vi "UNITEST MAIN v2.0.vi"() -> ()   [LabVIEW 2025] (continued)
    n868 = Close Reference(reference=w1021, error in (no error)=w1022) -> ()  [unwired: 1 out]
    n869 = Equal?(x=w1020, y=TRUE) -> (x = y?=w1018:bool)
    n870 = Select(t=i64 10 ("Period"), s=w1018, f=i64 100) -> (s? t:f=w1014:i64)
    n871 = Wait Until Next ms Multiple(millisecond multiple=w1014) -> ()  [unwired: 1 out]
  }
  n872 = timed-loop "Timed Loop" {
    shift-right: [w1107] -> _
    shift-left: w9 -> [w1108]
    tunnel: [w1101] -> w12
    tunnel: w41 -> [w1099]
    tunnel: w6 -> [w1098]
    tunnel: w10 -> [w1097]
    timing: w26 -> [_]
    timing-out: [_] -> w25
    shift-right: [w1095] -> _
    shift-left: w24 -> [w1096]
    shift-right: [w1093] -> _
    shift-left: w24 -> [w1094]
    shift-right: [w1091] -> _
    shift-left: w24 -> [w1092]
    shift-right: [w1090] -> _
    shift-left: w24 -> [w1089]
    stop <- w1106 stop-if-true
    # "Load Pid  Handling Loop"
    n873 = node-c288() -> ()  [unwired: 1 in, 1 out]
    n874 = call "Dequeue Message.vi"("error in (no error)"=w1098, "Message Queue"=w1099) -> ("error out"=w1105:errorcluster, "Message Data"=w1103:variant, "Message"=w1104:string, "dup Message Queue"=w1102:refnum<queue>)  [unwired: 6 in]
    n875 = case "Message Cases" shown="\"Load Pid Main\"" w1104 {
      selector: w1104 -> [_ _ _ _ _ w1216]
      tunnel: w1102 -> [w1115 w1144 _ w1195 w1211 _]
      tunnel: w1105 -> [w1118 w1142 w1188 w1199 w1205 _]
      tunnel: [w1119 w1145 w1182 w1197 w1207 w1217] -> w1100
      tunnel: w1108 -> [w1117 w1131 w1187 w1198 w1210 w1218]
      tunnel: [w1117 w1131 w1187 w1198 w1210 w1218] -> w1107
      tunnel: [_ _ _ _ TRUE _] -> w1106
      tunnel: w1103 -> [_ _ w1186 _ _ _]
      tunnel: w1097 -> [_ _ _ _ w1204 _]
      tunnel: w1096 -> [w1113 w1127 w1181 w1192 w1203 w1214]
      tunnel: [w1113 w1126 w1181 w1192 w1203 w1214] -> w1095
      tunnel: w1094 -> [w1114 w1125 w1180 w1191 w1202 w1215]
      tunnel: [w1114 w1124 w1180 w1191 w1202 w1215] -> w1093
      tunnel: w1092 -> [w1112 w1123 w1179 w1190 w1201 w1213]
      tunnel: [w1112 w1122 w1179 w1190 w1201 w1213] -> w1091
      tunnel: w1089 -> [_ w1121 _ _ _ _]
      tunnel: [w1111 w1120 w1178 w1189 w1200 w1212] -> w1090
      tunnel: w1089 -> [w1111 _ w1178 w1189 w1200 w1212]
      frame "init" {
        # "Initialize - All initialization work should take place in this message, since other loops can potentially enqueue messages that execute immediately after this one."
        n876 = call-poly "Enqueue Message.vi"("error in (no error)"=w1118, "Message"="Load Pid Main", "Message Queue"=w1115) -> ("error out"=w1119:errorcluster)  [unwired: 7 in, 1 out]
      }
      frame "Load Pid Main" {
        n877 = Unbundle By Name(w1131) -> ("Main Screen.Load En"=w1137:refnum<vi>)
        n878 = Unbundle By Name(w1131) -> ("PID.apply load"=w1132:refnum<vi>)
        n879 = property on="Property Node" class="Bool (strict)"(reference=w1137) -> (reference out=w1135:refnum<vi>, error out=w1136:errorcluster, "Value"=w1130:bool)  [unwired: 1 in]
        n880 = property on="Property Node" class="Bool (strict)"(reference=w1132) -> (reference out=w1134:refnum<vi>, error out=w1133:errorcluster, "Value"=w1129:bool)  [unwired: 1 in]
        n881 = Close Reference(reference=w1135, error in (no error)=w1136) -> ()  [unwired: 1 out]
        n882 = Close Reference(reference=w1134, error in (no error)=w1133) -> ()  [unwired: 1 out]
        n883 = Or(x=w1130, y=w1129) -> (x .or. y?=w1128:bool)
        n884 = case shown="True" w1128 {
          tunnel: w1142 -> [w1152 w1165]
          tunnel: [w1152 w1164] -> w1138
          tunnel: w1131 -> [_ w1163]
          tunnel: w1127 -> [w1151 w1162]
          tunnel: [w1151 w1161] -> w1126
          tunnel: w1125 -> [w1150 w1160]
          tunnel: [w1150 w1159] -> w1124
          tunnel: w1123 -> [w1147 w1156]
          tunnel: [w1147 w1155] -> w1122
          tunnel: w1121 -> [w1146 w1154]
          tunnel: [w1146 w1153] -> w1120
          frame False {
            n885 = local write "Checkbox 2"(TRUE ("Checkbox 2")) -> ()
            n886 = local write "Checkbox"(TRUE ("Checkbox")) -> ()
          }
          frame True {
            n887 = case shown="True" "Checkbox 2" {
              selector: "Checkbox 2" -> [_ w1168]
              tunnel: [FALSE ("Checkbox") "Checkbox"] -> w1158
              frame False {
              }
              frame True {
                n888 = Not(x=w1168) -> (.not. x?=w1167:bool)
                n889 = local write "Checkbox 2"(w1167) -> ()
              }
            }
            n890 = call "NEW LOAD CELL PID.vi"("filtered_load_in"=w1156, "filtered_deriv_in"=w1154, "integral_out"=w1160, "error in (no error)"=w1165, "prev_error_out"=w1162, "Checkbox"=w1158, "main ref"=w1163) -> ("error out"=w1164:errorcluster, "prev_error_out"=w1161:dbl, "integral_out"=w1159:dbl, "filtered_load_out"=w1155:dbl, "filtered_deriv_out"=w1153:dbl)
          }
        }
        n891 = Unbundle By Name(w1131) -> ("Main Home Screen.EXIT"=w1143:refnum<vi>)
        n892 = property on="Property Node" class="Bool (strict)"(reference=w1143) -> (reference out=w1140:refnum<vi>, error out=w1141:errorcluster, "Value"=w1139:bool)  [unwired: 1 in]
        n893 = case shown="False" w1139 {
          tunnel: [w1172 w1176] -> w1145
          tunnel: w1144 -> [w1171 w1175]
          tunnel: w1138 -> [w1170 w1174]
          frame True {
            n894 = call-poly "Enqueue Message.vi"("error in (no error)"=w1170, "Message"="Confirm Quit", "Message Queue"=w1171) -> ("error out"=w1172:errorcluster)  [unwired: 7 in, 1 out]
          }
          frame False {
            n895 = call-poly "Enqueue Message.vi"("error in (no error)"=w1174, "Message"="Load Pid Main", "Message Queue"=w1175) -> ("error out"=w1176:errorcluster)  [unwired: 7 in, 1 out]
          }
        }
        n896 = Close Reference(reference=w1140, error in (no error)=w1141) -> ()  [unwired: 1 out]
      }
      frame "Error" {
        # "#CodeRecommended - If you ever change the name of this \"Error\" message, you'll need to update the name in the Check Loop Error.vi as well."
        # "#CodeRecommended - Consider creating a system for logging errors in some way. These errors are for notification purposes only. Handling of specific errors should be performed in the message frames that generated the error."
        # "Error - Display an error dialog. This message is sent by the \"Error Handler\" VIs at the end of other loops in this application."
        n897 = Variant To Data(error in=w1188, type=errorcluster {"status"=FALSE, "code"=0, "source"=""} ("error constant"), Variant=w1186) -> (data=w1184:errorcluster, error out=w1183:errorcluster)
        n898 = call <vilib>:"Simple Error Handler.vi"("error in (no error)"=w1184) -> ()  [unwired: 4 in, 5 out]
        n899 = Merge Errors(w1183) -> (w1182:errorcluster)
      }
      frame "Confirm Quit" {
        # "#CodeNeeded - If you want to provide an \"Are you sure\" dialog (or some other notification) before the application exits, place that code here. This message is typically sent from a Panel Close? event."
        # "Confirm Quit - Message that can confirm whether or not the user wants to exit the application."
        n900 = call-poly "Enqueue Message.vi"("Priority Message? (F)"=TRUE, "error in (no error)"=w1199, "Message"="Exit", "Message Queue"=w1195) -> ("error out"=w1196:errorcluster)  [unwired: 6 in, 1 out]
        n901 = Merge Errors(w1196) -> (w1197:errorcluster)
      }
      frame "Exit" {
        # "Stop the VI"
        # "Release the message queue reference"
        # "#CodeNeeded - Add any required cleanup code here. Note that if 'Exit' was called as a result of an error, an error dialog will be displayed. Add any custom error handling for an 'Exit' condition here as well."
        # "Exit - Exit the application."
        n902 = call "Fire User Event - Stop.vi"("User Event - Stop"=w1204) -> ("error out"=w1206:errorcluster)  [unwired: 10 in]
        n903 = Release Queue(queue=w1211, error in (no error)=w1205) -> (error out=w1208:errorcluster)  [unwired: 1 in, 2 out]
        n904 = Merge Errors(w1206, w1208) -> (w1207:errorcluster)
      }
      frame Default {
        # "'Default' case only runs if there is a message that isn't defined in any of the other cases.  Output a programming error."
        n905 = xnode ("Error Ring")("parameter 0"=w1216) -> ("error out"=w1217:errorcluster)
      }
    }
    n906 = call "LAB-IQ Error Handler - Message Handling Loop.vi"("error in (no error)"=w1100, "Message Queue"=w1102) -> ("dup error in"=w1101:errorcluster)  [unwired: 8 in, 1 out]
    n907 = node-c288() -> ()  [unwired: 1 in, 1 out]
  }
  n908 = timed-loop {
    shift-right: [w1228] -> _
    shift-left: w9 -> [w1253]
    tunnel: [w1247] -> w5
    tunnel: w7 -> [w1245]
    tunnel: w6 -> [w1244]
    tunnel: w10 -> [w1243]
    timing: w4 -> [_]
    timing-out: [_] -> w3
    stop <- w1252 stop-if-true
    # "Acqoustic  Handling Loop"
    n909 = node-c288() -> ()  [unwired: 1 in, 1 out]
    n910 = call "Dequeue Message.vi"("error in (no error)"=w1244, "Message Queue"=w1245) -> ("error out"=w1251:errorcluster, "Message Data"=w1249:variant, "Message"=w1250:string, "dup Message Queue"=w1248:refnum<queue>)  [unwired: 6 in]
    n911 = case "Message Cases" shown="\"init\"" w1250 {
      selector: w1250 -> [_ _ _ _ _ w1350]
      tunnel: w1248 -> [w1268 w1283 _ w1337 w1349 _]
      tunnel: w1251 -> [w1262 w1274 w1334 w1341 w1343 _]
      tunnel: [w1270 w1284 w1328 w1339 w1345 w1351] -> w1246
      tunnel: w1253 -> [w1259 w1273 w1333 w1340 w1348 w1352]
      tunnel: [w1259 w1273 w1333 w1340 w1348 w1352] -> w1228
      tunnel: [_ _ _ _ TRUE _] -> w1252
      tunnel: w1249 -> [_ _ w1332 _ _ _]
      tunnel: w1243 -> [_ _ _ _ w1342 _]
      frame "init" {
        (unwired) dbl[] [] ("0UTPUT")
        # "Initialize - All initialization work should take place in this message, since other loops can potentially enqueue messages that execute immediately after this one."
        n912 = call "Acq Write Loop.vi"("Enum - Menu"=Write_Main_Enum."INIT", "error in (no error)"=w1262, "main ref"=w1259) -> ("error out"=w1267:errorcluster)  [unwired: 8 in]
        n913 = call <vilib>:"Clear Errors.vi"("error in (no error)"=w1267) -> ("error out"=w1266:errorcluster)  [unwired: 5 in, 1 out]
        n914 = call "Stall Data Flow.vim"("value in"=w1266, "milliseconds to wait"=u32 1000) -> ("value out"=w1265:errorcluster)  [unwired: 1 out]
        n915 = call "Acq Read Loop.vi"("Enum - Menu"=Read_Main_Enum."INIT", "error in (no error)"=w1265, "main ref"=w1259) -> ("error out"=w1263:errorcluster)  [unwired: 7 in, 1 out]
        n916 = call <vilib>:"Clear Errors.vi"("error in (no error)"=w1263) -> ("error out"=w1261:errorcluster)  [unwired: 5 in, 1 out]
        n917 = call-poly "Enqueue Message.vi"("error in (no error)"=w1261, "Message"="Acoustic Main", "Message Queue"=w1268) -> ("error out"=w1270:errorcluster)  [unwired: 7 in, 1 out]
      }
      frame "Acoustic Main" {
        n918 = Unbundle By Name(w1273) -> ("Environmental control.Acoustic Emission 3"=w1278:refnum<vi>)
        n919 = property on="Property Node" class="Bool (strict)"(reference=w1278) -> (reference out=w1276:refnum<vi>, error out=w1277:errorcluster, "Value"=w1275:bool)  [unwired: 1 in]
        n920 = Close Reference(reference=w1276, error in (no error)=w1277) -> ()  [unwired: 1 out]
        n921 = case shown="True" w1275 {
          tunnel: w1274 -> [w1285 w1315]
          tunnel: w1273 -> [_ w1287]
          tunnel: [w1285 w1307] -> w1272
          frame False {
          }
          frame True {
            n922 = call "Acq Read Loop.vi"("Enum - Menu"=Read_Main_Enum."READ", "error in (no error)"=w1315, "main ref"=w1287) -> ("error out"=w1313:errorcluster, "ERROR TEMP"=w1312:bool)  [unwired: 7 in]
            n923 = Unbundle By Name(w1287) -> ("Acquostic.Downlink Packet"=w1311:refnum<vi>)
            n924 = case shown="False" w1312 {
              tunnel: w1313 -> [w1316 w1319]
              tunnel: [w1316 w1318] -> w1308
              tunnel: w1287 -> [_ w1317]
              frame False {
              }
              frame True {
                n925 = call "Acoustic Reinitize.vi"("error in (no error)"=w1319, "Data Cluster"=w1317) -> ("error out"=w1318:errorcluster)  [unwired: 9 in]
              }
            }
            n926 = property on="Property Node" class="Clust (strict)"(reference=w1311, error in=w1308) -> (reference out=w1309:refnum<vi>, error out=w1310:errorcluster, "Value"=w1293:T8)
            n927 = Close Reference(reference=w1309, error in (no error)=w1310) -> (error out=w1307:errorcluster)
            n928 = Unbundle By Name(w1293) -> ("AE Ring-Down Counts"=w1291:u32)
            n929 = Unbundle By Name(w1293) -> ("Amplitude dB_AE"=w1292:sgl)
            n930 = Unbundle By Name(w1293) -> ("Peak Amplitude"=w1297:sgl)
            n931 = Unbundle By Name(w1293) -> ("Signal Energy"=w1286:sgl)
            n932 = Unbundle By Name(w1287) -> ("Main Screen.Acoustic Emission (mV)"=w1289:refnum<vi>)
            n933 = Unbundle By Name(w1287) -> ("Acquostic.Signal Energy"=w1306:refnum<vi>)
            n934 = Unbundle By Name(w1287) -> ("Acquostic.Amplitude db_AE"=w1301:refnum<vi>)
            n935 = Unbundle By Name(w1287) -> ("Acquostic.Peak Amplitude"=w1300:refnum<vi>)
            n936 = Unbundle By Name(w1287) -> ("Acquostic.AE Ring-Down Counts"=w1294:refnum<vi>)
            n937 = property class="DigNum (strict)"(reference=w1289, "Value"=w1286) -> (reference out=w1288:refnum<vi>, error out=w1290:errorcluster)  [unwired: 1 in]
            n938 = property on="Property Node" class="WFChart (strict)"(reference=w1306, "Value"=w1286) -> (reference out=w1304:refnum<vi>, error out=w1305:errorcluster)  [unwired: 1 in]
            n939 = property on="Property Node" class="WFChart (strict)"(reference=w1301, "Value"=w1292) -> (reference out=w1303:refnum<vi>, error out=w1302:errorcluster)  [unwired: 1 in]
            n940 = property on="Property Node" class="WFChart (strict)"(reference=w1300, "Value"=w1297) -> (reference out=w1298:refnum<vi>, error out=w1299:errorcluster)  [unwired: 1 in]
            n941 = property on="Property Node" class="WFChart (strict)"(reference=w1294, "Value"=w1291) -> (reference out=w1296:refnum<vi>, error out=w1295:errorcluster)  [unwired: 1 in]
            n942 = Close Reference(reference=w1288, error in (no error)=w1290) -> ()  [unwired: 1 out]
            n943 = Close Reference(reference=w1304, error in (no error)=w1305) -> ()  [unwired: 1 out]
            n944 = Close Reference(reference=w1303, error in (no error)=w1302) -> ()  [unwired: 1 out]
            n945 = Close Reference(reference=w1298, error in (no error)=w1299) -> ()  [unwired: 1 out]
            n946 = Close Reference(reference=w1296, error in (no error)=w1295) -> ()  [unwired: 1 out]
          }
        }
        n947 = Unbundle By Name(w1273) -> ("Main Home Screen.EXIT"=w1282:refnum<vi>)
        n948 = property on="Property Node" class="Bool (strict)"(reference=w1282) -> (reference out=w1280:refnum<vi>, error out=w1281:errorcluster, "Value"=w1279:bool)  [unwired: 1 in]
        n949 = call <vilib>:"Clear Errors.vi"("error in (no error)"=w1272) -> ("error out"=w1271:errorcluster)  [unwired: 5 in, 1 out]
        n950 = Close Reference(reference=w1280, error in (no error)=w1281) -> ()  [unwired: 1 out]
        n951 = case shown="False" w1279 {
          tunnel: [w1322 w1326] -> w1284
          tunnel: w1283 -> [w1321 w1325]
          tunnel: w1271 -> [w1320 w1324]
          frame True {
            n952 = call-poly "Enqueue Message.vi"("error in (no error)"=w1320, "Message"="Confirm Quit", "Message Queue"=w1321) -> ("error out"=w1322:errorcluster)  [unwired: 7 in, 1 out]
          }
          frame False {
            n953 = call-poly "Enqueue Message.vi"("error in (no error)"=w1324, "Message"="Acoustic Main", "Message Queue"=w1325) -> ("error out"=w1326:errorcluster)  [unwired: 7 in, 1 out]
          }
        }
      }
      frame "Error" {
        (unwired) dbl[] [] ("0UTPUT")
        # "#CodeRecommended - If you ever change the name of this \"Error\" message, you'll need to update the name in the Check Loop Error.vi as well."
        # "#CodeRecommended - Consider creating a system for logging errors in some way. These errors are for notification purposes only. Handling of specific errors should be performed in the message frames that generated the error."
        # "Error - Display an error dialog. This message is sent by the \"Error Handler\" VIs at the end of other loops in this application."
        n954 = Variant To Data(error in=w1334, type=errorcluster {"status"=FALSE, "code"=0, "source"=""} ("error constant"), Variant=w1332) -> (data=w1330:errorcluster, error out=w1329:errorcluster)
        n955 = call <vilib>:"Simple Error Handler.vi"("error in (no error)"=w1330) -> ()  [unwired: 4 in, 5 out]
        n956 = Merge Errors(w1329) -> (w1328:errorcluster)
      }
      frame "Confirm Quit" {
        (unwired) dbl[] [] ("0UTPUT")
        # "#CodeNeeded - If you want to provide an \"Are you sure\" dialog (or some other notification) before the application exits, place that code here. This message is typically sent from a Panel Close? event."
        # "Confirm Quit - Message that can confirm whether or not the user wants to exit the application."
        n957 = call-poly "Enqueue Message.vi"("Priority Message? (F)"=TRUE, "error in (no error)"=w1341, "Message"="Exit", "Message Queue"=w1337) -> ("error out"=w1338:errorcluster)  [unwired: 6 in, 1 out]
        n958 = Merge Errors(w1338) -> (w1339:errorcluster)
      }
      frame "Exit" {
        (unwired) dbl[] [] ("0UTPUT")
        # "Stop the VI"
        # "Release the message queue reference"
        # "#CodeNeeded - Add any required cleanup code here. Note that if 'Exit' was called as a result of an error, an error dialog will be displayed. Add any custom error handling for an 'Exit' condition here as well."
        # "Exit - Exit the application."
        n959 = call "Fire User Event - Stop.vi"("User Event - Stop"=w1342) -> ("error out"=w1344:errorcluster)  [unwired: 10 in]
        n960 = Release Queue(queue=w1349, error in (no error)=w1343) -> (error out=w1346:errorcluster)  [unwired: 1 in, 2 out]
        n961 = Merge Errors(w1344, w1346) -> (w1345:errorcluster)
      }
      frame Default {
        # "'Default' case only runs if there is a message that isn't defined in any of the other cases.  Output a programming error."
        n962 = xnode ("Error Ring")("parameter 0"=w1350) -> ("error out"=w1351:errorcluster)
      }
    }
    n963 = Unbundle By Name(w1228) -> ("Environmental control.Acoustic Emission 3"=w1242:refnum<vi>)
    n964 = call "LAB-IQ Error Handler - Message Handling Loop.vi"("error in (no error)"=w1246, "Message Queue"=w1248) -> ("dup error in"=w1247:errorcluster)  [unwired: 8 in, 1 out]
    n965 = Unbundle By Name(w1228) -> ("Motion Module.Scratch"=w1229:refnum<vi>)
    n966 = property on="Property Node" class="Bool (strict)"(reference=w1242) -> (reference out=w1240:refnum<vi>, error out=w1241:errorcluster, "Value"=w1239:bool)  [unwired: 1 in]
    n967 = property on="Property Node" class="Bool (strict)"(reference=w1229) -> (reference out=w1231:refnum<vi>, error out=w1230:errorcluster, "Value"=w1232:bool)  [unwired: 1 in]
    n968 = Close Reference(reference=w1240, error in (no error)=w1241) -> ()  [unwired: 1 out]
    n969 = Equal?(x=w1239, y=TRUE) -> (x = y?=w1237:bool)
    n970 = Close Reference(reference=w1231, error in (no error)=w1230) -> ()  [unwired: 1 out]
    n971 = Equal?(x=w1232, y=TRUE) -> (x = y?=w1226:bool)
    n972 = And(x=w1237, y=w1226) -> (x .and. y?=w1227:bool)
    n973 = Select(t=i64 5 ("Period"), s=w1227, f=i64 1000) -> (s? t:f=w1234:i64)
    n974 = node-c288(w1234) -> ()  [unwired: 1 in, 1 out]
  }
  n975 = disable-structure "Diagram Disable Structure" shown="Disabled" {
    disable-tunnel: w48 -> [w1364 _]
    disable-tunnel: w9 -> [w1363 _]
    disable-tunnel: w10 -> [w1362 _]
    disable-tunnel: w6 -> [w1361 w1430]
    disable-tunnel: [w1360 w1430] -> w32
    frame Disabled {
      n976 = while {
        shift-right: [w1375] -> _
        shift-left: w1363 -> [w1376]
        tunnel: [w1369] -> w1360
        tunnel: w1364 -> [w1367]
        tunnel: w1361 -> [w1366]
        tunnel: w1362 -> [w1365]
        stop <- w1374 stop-if-true
        # "Temperature  Handling Loop"
        n977 = call "Dequeue Message.vi"("error in (no error)"=w1366, "Message Queue"=w1367) -> ("error out"=w1373:errorcluster, "Message Data"=w1371:variant, "Message"=w1372:string, "dup Message Queue"=w1370:refnum<queue>)  [unwired: 6 in]
        n978 = case "Message Cases" shown="\"Temperature Main\"" w1372 {
          selector: w1372 -> [_ _ _ _ _ w1420]
          tunnel: w1370 -> [w1377 w1388 _ w1407 w1419 _]
          tunnel: w1373 -> [w1380 w1385 w1404 w1411 w1413 _]
          tunnel: [w1381 w1389 w1398 w1409 w1415 w1421] -> w1368
          tunnel: w1376 -> [w1379 w1387 w1403 w1410 w1418 w1422]
          tunnel: [w1379 w1387 w1403 w1410 w1418 w1422] -> w1375
          tunnel: [_ _ _ _ TRUE _] -> w1374
          tunnel: w1371 -> [_ _ w1402 _ _ _]
          tunnel: w1365 -> [_ _ _ _ w1412 _]
          frame "init" {
            # "Initialize - All initialization work should take place in this message, since other loops can potentially enqueue messages that execute immediately after this one."
            n979 = call-poly "Enqueue Message.vi"("error in (no error)"=w1380, "Message"="Temperature Main", "Message Queue"=w1377) -> ("error out"=w1381:errorcluster)  [unwired: 7 in, 1 out]
          }
          frame "Temperature Main" {
            n980 = Unbundle By Name(w1387) -> ("Main Home Screen.EXIT"=w1386:refnum<vi>)
            n981 = property on="Property Node" class="Bool (strict)"(reference=w1386) -> (reference out=w1383:refnum<vi>, error out=w1384:errorcluster, "Value"=w1382:bool)  [unwired: 1 in]
            n982 = case shown="False" w1382 {
              tunnel: [w1392 w1396] -> w1389
              tunnel: w1388 -> [w1391 w1395]
              tunnel: w1385 -> [w1390 w1394]
              frame True {
                n983 = call-poly "Enqueue Message.vi"("error in (no error)"=w1390, "Message"="Confirm Quit", "Message Queue"=w1391) -> ("error out"=w1392:errorcluster)  [unwired: 7 in, 1 out]
              }
              frame False {
                n984 = call-poly "Enqueue Message.vi"("error in (no error)"=w1394, "Message"="Temperature Main", "Message Queue"=w1395) -> ("error out"=w1396:errorcluster)  [unwired: 7 in, 1 out]
              }
            }
            n985 = Close Reference(reference=w1383, error in (no error)=w1384) -> ()  [unwired: 1 out]
          }
          frame "Error" {
            # "#CodeRecommended - If you ever change the name of this \"Error\" message, you'll need to update the name in the Check Loop Error.vi as well."
            # "#CodeRecommended - Consider creating a system for logging errors in some way. These errors are for notification purposes only. Handling of specific errors should be performed in the message frames that generated the error."
            # "Error - Display an error dialog. This message is sent by the \"Error Handler\" VIs at the end of other loops in this application."
            n986 = Variant To Data(error in=w1404, type=errorcluster {"status"=FALSE, "code"=0, "source"=""} ("error constant"), Variant=w1402) -> (data=w1400:errorcluster, error out=w1399:errorcluster)
            n987 = call <vilib>:"Simple Error Handler.vi"("error in (no error)"=w1400) -> ()  [unwired: 4 in, 5 out]
            n988 = Merge Errors(w1399) -> (w1398:errorcluster)
          }
          frame "Confirm Quit" {
            # "#CodeNeeded - If you want to provide an \"Are you sure\" dialog (or some other notification) before the application exits, place that code here. This message is typically sent from a Panel Close? event."
            # "Confirm Quit - Message that can confirm whether or not the user wants to exit the application."
            n989 = call-poly "Enqueue Message.vi"("Priority Message? (F)"=TRUE, "error in (no error)"=w1411, "Message"="Exit", "Message Queue"=w1407) -> ("error out"=w1408:errorcluster)  [unwired: 6 in, 1 out]
            n990 = Merge Errors(w1408) -> (w1409:errorcluster)
          }
          frame "Exit" {
            # "Stop the VI"
            # "Release the message queue reference"
            # "#CodeNeeded - Add any required cleanup code here. Note that if 'Exit' was called as a result of an error, an error dialog will be displayed. Add any custom error handling for an 'Exit' condition here as well."
            # "Exit - Exit the application."
            n991 = call "Fire User Event - Stop.vi"("User Event - Stop"=w1412) -> ("error out"=w1414:errorcluster)  [unwired: 10 in]
            n992 = Release Queue(queue=w1419, error in (no error)=w1413) -> (error out=w1416:errorcluster)  [unwired: 1 in, 2 out]
            n993 = Merge Errors(w1414, w1416) -> (w1415:errorcluster)
          }
          frame Default {
            # "'Default' case only runs if there is a message that isn't defined in any of the other cases.  Output a programming error."
            n994 = xnode ("Error Ring")("parameter 0"=w1420) -> ("error out"=w1421:errorcluster)
          }
        }
        n995 = call "LAB-IQ Error Handler - Message Handling Loop.vi"("error in (no error)"=w1368, "Message Queue"=w1370) -> ("dup error in"=w1369:errorcluster)  [unwired: 8 in, 1 out]
      }
    }
    frame Enabled {
    }
  }
  n996 = while {
    tunnel: w78 -> [w1438]
    shift-right: [w1436] -> w75
    shift-left: w72 -> [w1437]
    tunnel: [w1432] -> w73
    stop <- w1434 stop-if-true
    # "Event Handling Loop"
    n997 = event shown="[1] Timeout" {
      selector: w1437 -> [_ _ _ _ _ _ _ _ _ _ _ _ _ _ _ _ _ _ _ _ _ _ _ _ _ _ _ _ _ _ _ _ _ _ _ _ _ _ _ _ _ _ _ _ _ _ _ _ _ _ _ _ _ _ _ _ _ _ _ _ _ _ _ _ _ _ _ _ _ _ _ _ _ _ _ _ _ _ _]
      dyn-events: [_ _ _ _ _ _ _ _ _ _ _ _ _ _ _ _ _ _ _ _ _ _ _ _ _ _ _ _ _ _ _ _ _ _ _ _ _ _ _ _ _ _ _ _ _ _ _ _ _ _ _ _ _ _ _ _ _ _ _ _ _ _ _ _ _ _ _ _ _ _ _ _ _ _ _ _ _ _ _] -> w1436
      timeout: 100 -> [_ _ _ _ _ _ _ _ _ _ _ _ _ _ _ _ _ _ _ _ _ _ _ _ _ _ _ _ _ _ _ _ _ _ _ _ _ _ _ _ _ _ _ _ _ _ _ _ _ _ _ _ _ _ _ _ _ _ _ _ _ _ _ _ _ _ _ _ _ _ _ _ _ _ _ _ _ _ _]
      tunnel: [_ _ _ _ _ _ _ _ _ _ _ _ _ _ _ _ _ _ _ _ _ _ _ _ _ _ _ _ _ _ _ _ _ _ _ _ _ _ _ _ _ _ _ _ _ _ _ _ _ _ _ _ _ _ _ _ _ _ _ _ _ _ _ _ _ _ _ _ _ _ _ _ _ _ _ _ _ _ TRUE ("Discard?")] -> w1434
      tunnel: w1438 -> [w1443 w1449 w1452 w1457 w1462 w1467 w1472 w1477 w1482 w1487 w1492 w1497 w1502 w1507 w1512 w1517 w1522 w1527 w1532 w1537 w1542 w1547 w1552 w1557 w1562 w1567 w1572 w1577 w1582 w1587 w1592 w1597 w1602 w1607 w1612 w1617 w1622 w1627 w1632 w1637 w1642 w1647 w1652 w1657 w1662 w1667 w1672 w1677 w1682 w1687 w1692 w1697 w1702 w1707 w1712 w1717 w1722 w1727 w1732 w1737 w1742 w1747 w1752 w1757 w1762 w1767 w1772 w1777 w1782 w1787 w1792 w1797 w1802 w1807 w1812 w1817 w1820 w1825 w1827]
      tunnel: [w1442 w1448 w1450 w1455 w1460 w1465 w1470 w1475 w1480 w1485 w1490 w1495 w1500 w1505 w1510 w1515 w1520 w1525 w1530 w1535 w1540 w1545 w1550 w1555 w1560 w1565 w1570 w1575 w1580 w1585 w1590 w1595 w1600 w1605 w1610 w1615 w1620 w1625 w1630 w1635 w1640 w1645 w1650 w1655 w1660 w1665 w1670 w1675 w1680 w1685 w1690 w1695 w1700 w1705 w1710 w1715 w1720 w1725 w1730 w1735 w1740 w1745 w1750 w1755 w1760 w1765 w1770 w1775 w1780 w1785 w1790 w1795 w1800 w1805 w1810 w1815 _ w1824 _] -> w1435
      tunnel: [w1441 w1447 w1451 w1456 w1461 w1466 w1471 w1476 w1481 w1486 w1491 w1496 w1501 w1506 w1511 w1516 w1521 w1526 w1531 w1536 w1541 w1546 w1551 w1556 w1561 w1566 w1571 w1576 w1581 w1586 w1591 w1596 w1601 w1606 w1611 w1616 w1621 w1626 w1631 w1636 w1641 w1646 w1651 w1656 w1661 w1666 w1671 w1676 w1681 w1686 w1691 w1696 w1701 w1706 w1711 w1716 w1721 w1726 w1731 w1736 w1741 w1746 w1751 w1756 w1761 w1766 w1771 w1776 w1781 w1786 w1791 w1796 w1801 w1806 w1811 w1816 w1820 w1823 w1827] -> w1433
      event Panel Close? {
        n998 = event-data() -> ()  [unwired: 1 in, 1 out]
        n999 = call-poly "Enqueue Message.vi"("Priority Message? (F)"=TRUE, "Message"="Confirm Quit", "Message Queue"=w1443) -> ("error out"=w1442:errorcluster, "dup Message Queue"=w1441:refnum<queue>)  [unwired: 7 in]
        n1000 = event-data ("Event Filter Node")("Discard?"=TRUE) -> ()  [unwired: 1 in, 1 out]
      }
      event Timeout {
        n1001 = event-data() -> ()  [unwired: 1 in, 1 out]
        n1002 = call-poly "Enqueue Message.vi"("Priority Message? (F)"=TRUE, "Message"="Timeout", "Message Queue"=w1449) -> ("error out"=w1448:errorcluster, "dup Message Queue"=w1447:refnum<queue>)  [unwired: 7 in]
      }
      event "SAVE  2": Value Change {
        n1003 = event-data() -> ()  [unwired: 1 in, 1 out]
        n1004 = call-poly "Enqueue Message.vi"("Priority Message? (F)"=TRUE, "Message"="Service Save", "Message Queue"=w1452) -> ("error out"=w1450:errorcluster, "dup Message Queue"=w1451:refnum<queue>)  [unwired: 7 in]
      }
      event "Home": Value Change {
        n1005 = event-data() -> ()  [unwired: 1 in, 1 out]
        n1006 = call-poly "Enqueue Message.vi"("Priority Message? (F)"=TRUE, "Message"="HOME", "Message Queue"=w1457) -> ("error out"=w1455:errorcluster, "dup Message Queue"=w1456:refnum<queue>)  [unwired: 7 in]
      }
      event "Platform Settings": Value Change {
        n1007 = event-data() -> ()  [unwired: 1 in, 1 out]
        n1008 = call-poly "Enqueue Message.vi"("Priority Message? (F)"=TRUE, "Message"="Platform Setting", "Message Queue"=w1462) -> ("error out"=w1460:errorcluster, "dup Message Queue"=w1461:refnum<queue>)  [unwired: 7 in]
      }
      event "Configure": Value Change {
        n1009 = event-data() -> ()  [unwired: 1 in, 1 out]
        n1010 = call-poly "Enqueue Message.vi"("Priority Message? (F)"=TRUE, "Message"="Configure", "Message Queue"=w1467) -> ("error out"=w1465:errorcluster, "dup Message Queue"=w1466:refnum<queue>)  [unwired: 7 in]
      }
      event "Analysis": Value Change {
        n1011 = event-data() -> ()  [unwired: 1 in, 1 out]
        n1012 = call-poly "Enqueue Message.vi"("Priority Message? (F)"=TRUE, "Message"="Analysis", "Message Queue"=w1472) -> ("error out"=w1470:errorcluster, "dup Message Queue"=w1471:refnum<queue>)  [unwired: 7 in]
      }
      event "service 2": Value Change {
        n1013 = event-data() -> ()  [unwired: 1 in, 1 out]
        n1014 = call-poly "Enqueue Message.vi"("Priority Message? (F)"=TRUE, "Message"="service 2", "Message Queue"=w1477) -> ("error out"=w1475:errorcluster, "dup Message Queue"=w1476:refnum<queue>)  [unwired: 7 in]
      }
      event "Auto": Value Change {
        n1015 = event-data() -> ()  [unwired: 1 in, 1 out]
        n1016 = call-poly "Enqueue Message.vi"("Priority Message? (F)"=TRUE, "Message"="Auto", "Message Queue"=w1482) -> ("error out"=w1480:errorcluster, "dup Message Queue"=w1481:refnum<queue>)  [unwired: 7 in]
      }
      event "Select Load Head": Value Change {
        n1017 = event-data() -> ()  [unwired: 1 in, 1 out]
        n1018 = call-poly "Enqueue Message.vi"("Priority Message? (F)"=TRUE, "Message"="Select Load Head", "Message Queue"=w1487) -> ("error out"=w1485:errorcluster, "dup Message Queue"=w1486:refnum<queue>)  [unwired: 7 in]
      }
      event "com 3": Value Change {
        n1019 = event-data() -> ()  [unwired: 1 in, 1 out]
        n1020 = call-poly "Enqueue Message.vi"("Priority Message? (F)"=TRUE, "Message"="com 3", "Message Queue"=w1492) -> ("error out"=w1490:errorcluster, "dup Message Queue"=w1491:refnum<queue>)  [unwired: 7 in]
      }
      event "Loading Mode": Value Change {
        n1021 = event-data() -> ()  [unwired: 1 in, 1 out]
        n1022 = call-poly "Enqueue Message.vi"("Priority Message? (F)"=TRUE, "Message"="Loading Mode", "Message Queue"=w1497) -> ("error out"=w1495:errorcluster, "dup Message Queue"=w1496:refnum<queue>)  [unwired: 7 in]
      }
      event "SSP 0.3": Value Change {
        n1023 = event-data() -> ()  [unwired: 1 in, 1 out]
        n1024 = call-poly "Enqueue Message.vi"("Priority Message? (F)"=TRUE, "Message"="SSP 0.3", "Message Queue"=w1502) -> ("error out"=w1500:errorcluster, "dup Message Queue"=w1501:refnum<queue>)  [unwired: 7 in]
      }
      event "SSP 0.5": Value Change {
        n1025 = event-data() -> ()  [unwired: 1 in, 1 out]
        n1026 = call-poly "Enqueue Message.vi"("Priority Message? (F)"=TRUE, "Message"="SSP 0.5", "Message Queue"=w1507) -> ("error out"=w1505:errorcluster, "dup Message Queue"=w1506:refnum<queue>)  [unwired: 7 in]
      }
      event "SSP 0.75": Value Change {
        n1027 = event-data() -> ()  [unwired: 1 in, 1 out]
        n1028 = call-poly "Enqueue Message.vi"("Priority Message? (F)"=TRUE, "Message"="SSP 0.75", "Message Queue"=w1512) -> ("error out"=w1510:errorcluster, "dup Message Queue"=w1511:refnum<queue>)  [unwired: 7 in]
      }
      event "LHBack": Value Change {
        n1029 = event-data() -> ()  [unwired: 1 in, 1 out]
        n1030 = call-poly "Enqueue Message.vi"("Priority Message? (F)"=TRUE, "Message"="LHBack", "Message Queue"=w1517) -> ("error out"=w1515:errorcluster, "dup Message Queue"=w1516:refnum<queue>)  [unwired: 7 in]
      }
      event "LHNext": Value Change {
        n1031 = event-data() -> ()  [unwired: 1 in, 1 out]
        n1032 = call-poly "Enqueue Message.vi"("Priority Message? (F)"=TRUE, "Message"="LHNext", "Message Queue"=w1522) -> ("error out"=w1520:errorcluster, "dup Message Queue"=w1521:refnum<queue>)  [unwired: 7 in]
      }
      event "Rot Ver": Value Change {
        n1033 = event-data() -> ()  [unwired: 1 in, 1 out]
        n1034 = call-poly "Enqueue Message.vi"("Priority Message? (F)"=TRUE, "Message"="Rot Ver", "Message Queue"=w1527) -> ("error out"=w1525:errorcluster, "dup Message Queue"=w1526:refnum<queue>)  [unwired: 7 in]
      }
      event "Traction": Value Change {
        n1035 = event-data() -> ()  [unwired: 1 in, 1 out]
        n1036 = call-poly "Enqueue Message.vi"("Priority Message? (F)"=TRUE, "Message"="Traction", "Message Queue"=w1532) -> ("error out"=w1530:errorcluster, "dup Message Queue"=w1531:refnum<queue>)  [unwired: 7 in]
      }
      event "Scratch": Value Change {
        n1037 = event-data() -> ()  [unwired: 1 in, 1 out]
        n1038 = call-poly "Enqueue Message.vi"("Priority Message? (F)"=TRUE, "Message"="Scratch", "Message Queue"=w1537) -> ("error out"=w1535:errorcluster, "dup Message Queue"=w1536:refnum<queue>)  [unwired: 7 in]
      }
      event "Motion Mode:": Value Change {
        n1039 = event-data() -> ()  [unwired: 1 in, 1 out]
        n1040 = call-poly "Enqueue Message.vi"("Priority Message? (F)"=TRUE, "Message"="Motion Mode:", "Message Queue"=w1542) -> ("error out"=w1540:errorcluster, "dup Message Queue"=w1541:refnum<queue>)  [unwired: 7 in]
      }
      event "MMBack": Value Change {
        n1041 = event-data() -> ()  [unwired: 1 in, 1 out]
        n1042 = call-poly "Enqueue Message.vi"("Priority Message? (F)"=TRUE, "Message"="MMBack", "Message Queue"=w1547) -> ("error out"=w1545:errorcluster, "dup Message Queue"=w1546:refnum<queue>)  [unwired: 7 in]
      }
      event "MMNext": Value Change {
        n1043 = event-data() -> ()  [unwired: 1 in, 1 out]
        n1044 = call-poly "Enqueue Message.vi"("Priority Message? (F)"=TRUE, "Message"="MMNext", "Message Queue"=w1552) -> ("error out"=w1550:errorcluster, "dup Message Queue"=w1551:refnum<queue>)  [unwired: 7 in]
      }
      event "APBack": Value Change {
        n1045 = event-data() -> ()  [unwired: 1 in, 1 out]
        n1046 = call-poly "Enqueue Message.vi"("Priority Message? (F)"=TRUE, "Message"="APBack", "Message Queue"=w1557) -> ("error out"=w1555:errorcluster, "dup Message Queue"=w1556:refnum<queue>)  [unwired: 7 in]
      }
      event "SNext": Value Change {
        n1047 = event-data() -> ()  [unwired: 1 in, 1 out]
        n1048 = call-poly "Enqueue Message.vi"("Priority Message? (F)"=TRUE, "Message"="SNext", "Message Queue"=w1562) -> ("error out"=w1560:errorcluster, "dup Message Queue"=w1561:refnum<queue>)  [unwired: 7 in]
      }
      event "ZeroAll": Value Change {
        n1049 = event-data() -> ()  [unwired: 1 in, 1 out]
        n1050 = call-poly "Enqueue Message.vi"("Priority Message? (F)"=TRUE, "Message"="ZeroAll", "Message Queue"=w1567) -> ("error out"=w1565:errorcluster, "dup Message Queue"=w1566:refnum<queue>)  [unwired: 7 in]
      }
      event "Enable Platform": Value Change {
        n1051 = event-data() -> ()  [unwired: 1 in, 1 out]
        n1052 = call-poly "Enqueue Message.vi"("Priority Message? (F)"=TRUE, "Message"="Enable Platform", "Message Queue"=w1572) -> ("error out"=w1570:errorcluster, "dup Message Queue"=w1571:refnum<queue>)  [unwired: 7 in]
      }
      event "Heave Up main": Value Change {
        n1053 = event-data() -> ()  [unwired: 1 in, 1 out]
        n1054 = call-poly "Enqueue Message.vi"("Priority Message? (F)"=TRUE, "Message"="Heave Up main", "Message Queue"=w1577) -> ("error out"=w1575:errorcluster, "dup Message Queue"=w1576:refnum<queue>)  [unwired: 7 in]
      }
      event "Heave Up MM": Value Change {
        n1055 = event-data() -> ()  [unwired: 1 in, 1 out]
        n1056 = call-poly "Enqueue Message.vi"("Priority Message? (F)"=TRUE, "Message"="Heave Up MM", "Message Queue"=w1582) -> ("error out"=w1580:errorcluster, "dup Message Queue"=w1581:refnum<queue>)  [unwired: 7 in]
      }
      event "Heave Down Main": Value Change {
        n1057 = event-data() -> ()  [unwired: 1 in, 1 out]
        n1058 = call-poly "Enqueue Message.vi"("Priority Message? (F)"=TRUE, "Message"="Heave Down Main", "Message Queue"=w1587) -> ("error out"=w1585:errorcluster, "dup Message Queue"=w1586:refnum<queue>)  [unwired: 7 in]
      }
      event "Heave Down MM": Value Change {
        n1059 = event-data() -> ()  [unwired: 1 in, 1 out]
        n1060 = call-poly "Enqueue Message.vi"("Priority Message? (F)"=TRUE, "Message"="Heave Down MM", "Message Queue"=w1592) -> ("error out"=w1590:errorcluster, "dup Message Queue"=w1591:refnum<queue>)  [unwired: 7 in]
      }
      event "Manual Write Heave & Surge": Value Change {
        n1061 = event-data() -> ()  [unwired: 1 in, 1 out]
        n1062 = call-poly "Enqueue Message.vi"("Priority Message? (F)"=TRUE, "Message"="Manual Write Heave & Surge", "Message Queue"=w1597) -> ("error out"=w1595:errorcluster, "dup Message Queue"=w1596:refnum<queue>)  [unwired: 7 in]
      }
      event "Manual Write SWAY": Value Change {
        n1063 = event-data() -> ()  [unwired: 1 in, 1 out]
        n1064 = call-poly "Enqueue Message.vi"("Priority Message? (F)"=TRUE, "Message"="Manual Write SWAY", "Message Queue"=w1602) -> ("error out"=w1600:errorcluster, "dup Message Queue"=w1601:refnum<queue>)  [unwired: 7 in]
      }
      event "Surge Backward Main": Value Change {
        n1065 = event-data() -> ()  [unwired: 1 in, 1 out]
        n1066 = call-poly "Enqueue Message.vi"("Priority Message? (F)"=TRUE, "Message"="Surge Backward Main", "Message Queue"=w1607) -> ("error out"=w1605:errorcluster, "dup Message Queue"=w1606:refnum<queue>)  [unwired: 7 in]
      }
      event "Surge Backward MM": Value Change {
        n1067 = event-data() -> ()  [unwired: 1 in, 1 out]
        n1068 = call-poly "Enqueue Message.vi"("Priority Message? (F)"=TRUE, "Message"="Surge Backward MM", "Message Queue"=w1612) -> ("error out"=w1610:errorcluster, "dup Message Queue"=w1611:refnum<queue>)  [unwired: 7 in]
      }
      event "Surge Forward Main": Value Change {
        n1069 = event-data() -> ()  [unwired: 1 in, 1 out]
        n1070 = call-poly "Enqueue Message.vi"("Priority Message? (F)"=TRUE, "Message"="Surge Forward Main", "Message Queue"=w1617) -> ("error out"=w1615:errorcluster, "dup Message Queue"=w1616:refnum<queue>)  [unwired: 7 in]
      }
      event "Surge Forward MM": Value Change {
        n1071 = event-data() -> ()  [unwired: 1 in, 1 out]
        n1072 = call-poly "Enqueue Message.vi"("Priority Message? (F)"=TRUE, "Message"="Surge Forward MM", "Message Queue"=w1622) -> ("error out"=w1620:errorcluster, "dup Message Queue"=w1621:refnum<queue>)  [unwired: 7 in]
      }
      event "Sway Left Main": Value Change {
        n1073 = event-data() -> ()  [unwired: 1 in, 1 out]
        n1074 = call-poly "Enqueue Message.vi"("Priority Message? (F)"=TRUE, "Message"="Sway Left Main", "Message Queue"=w1627) -> ("error out"=w1625:errorcluster, "dup Message Queue"=w1626:refnum<queue>)  [unwired: 7 in]
      }
      event "Sway Left MM": Value Change {
        n1075 = event-data() -> ()  [unwired: 1 in, 1 out]
        n1076 = call-poly "Enqueue Message.vi"("Priority Message? (F)"=TRUE, "Message"="Sway Left MM", "Message Queue"=w1632) -> ("error out"=w1630:errorcluster, "dup Message Queue"=w1631:refnum<queue>)  [unwired: 7 in]
      }
      event "Sway Right MM": Value Change {
        n1077 = event-data() -> ()  [unwired: 1 in, 1 out]
        n1078 = call-poly "Enqueue Message.vi"("Priority Message? (F)"=TRUE, "Message"="Sway Right MM", "Message Queue"=w1637) -> ("error out"=w1635:errorcluster, "dup Message Queue"=w1636:refnum<queue>)  [unwired: 7 in]
      }
      event "Sway Right Main": Value Change {
        n1079 = event-data() -> ()  [unwired: 1 in, 1 out]
        n1080 = call-poly "Enqueue Message.vi"("Priority Message? (F)"=TRUE, "Message"="Sway Right Main", "Message Queue"=w1642) -> ("error out"=w1640:errorcluster, "dup Message Queue"=w1641:refnum<queue>)  [unwired: 7 in]
      }
      event "Load En": Value Change {
        n1081 = event-data() -> ()  [unwired: 1 in, 1 out]
        n1082 = call-poly "Enqueue Message.vi"("Priority Message? (F)"=TRUE, "Message"="Load En", "Message Queue"=w1647) -> ("error out"=w1645:errorcluster, "dup Message Queue"=w1646:refnum<queue>)  [unwired: 7 in]
      }
      event "PID.apply load": Value Change {
        n1083 = event-data() -> ()  [unwired: 1 in, 1 out]
        n1084 = call-poly "Enqueue Message.vi"("Priority Message? (F)"=TRUE, "Message"="apply load", "Message Queue"=w1652) -> ("error out"=w1650:errorcluster, "dup Message Queue"=w1651:refnum<queue>)  [unwired: 7 in]
      }
      event "BACK": Value Change {
        n1085 = event-data() -> ()  [unwired: 1 in, 1 out]
        n1086 = call-poly "Enqueue Message.vi"("Priority Message? (F)"=TRUE, "Message"="BACK", "Message Queue"=w1657) -> ("error out"=w1655:errorcluster, "dup Message Queue"=w1656:refnum<queue>)  [unwired: 7 in]
      }
      event "Start Test": Value Change {
        n1087 = event-data() -> ()  [unwired: 1 in, 1 out]
        n1088 = call-poly "Enqueue Message.vi"("Priority Message? (F)"=TRUE, "Message"="Start Test", "Message Queue"=w1662) -> ("error out"=w1660:errorcluster, "dup Message Queue"=w1661:refnum<queue>)  [unwired: 7 in]
      }
      event "STOP": Value Change {
        n1089 = event-data() -> ()  [unwired: 1 in, 1 out]
        n1090 = call-poly "Enqueue Message.vi"("Priority Message? (F)"=TRUE, "Message"="STOP", "Message Queue"=w1667) -> ("error out"=w1665:errorcluster, "dup Message Queue"=w1666:refnum<queue>)  [unwired: 7 in]
      }
      event "PlaceModule": Value Change {
        n1091 = event-data() -> ()  [unwired: 1 in, 1 out]
        n1092 = call-poly "Enqueue Message.vi"("Priority Message? (F)"=TRUE, "Message"="PlaceModule", "Message Queue"=w1672) -> ("error out"=w1670:errorcluster, "dup Message Queue"=w1671:refnum<queue>)  [unwired: 7 in]
      }
      event "HomeRot", "HomeScratch", "HomeScratch": Value Change {
        n1093 = event-data() -> ()  [unwired: 1 in, 1 out]
        n1094 = call-poly "Enqueue Message.vi"("Priority Message? (F)"=TRUE, "Message"="Stage Homing", "Message Queue"=w1677) -> ("error out"=w1675:errorcluster, "dup Message Queue"=w1676:refnum<queue>)  [unwired: 7 in]
      }
      event "Clear 3": Value Change {
        n1095 = event-data() -> ()  [unwired: 1 in, 1 out]
        n1096 = call-poly "Enqueue Message.vi"("Priority Message? (F)"=TRUE, "Message"="Clear 3", "Message Queue"=w1682) -> ("error out"=w1680:errorcluster, "dup Message Queue"=w1681:refnum<queue>)  [unwired: 7 in]
      }
      event "Set WTD": Value Change {
        n1097 = event-data() -> ()  [unwired: 1 in, 1 out]
        n1098 = call-poly "Enqueue Message.vi"("Priority Message? (F)"=TRUE, "Message"="Set WTD", "Message Queue"=w1687) -> ("error out"=w1685:errorcluster, "dup Message Queue"=w1686:refnum<queue>)  [unwired: 7 in]
      }
      event "Import 2": Value Change {
        n1099 = event-data() -> ()  [unwired: 1 in, 1 out]
        n1100 = call-poly "Enqueue Message.vi"("Priority Message? (F)"=TRUE, "Message"="Import 2", "Message Queue"=w1692) -> ("error out"=w1690:errorcluster, "dup Message Queue"=w1691:refnum<queue>)  [unwired: 7 in]
      }
      event "Save 2": Value Change {
        n1101 = event-data() -> ()  [unwired: 1 in, 1 out]
        n1102 = call-poly "Enqueue Message.vi"("Priority Message? (F)"=TRUE, "Message"="Save 2", "Message Queue"=w1697) -> ("error out"=w1695:errorcluster, "dup Message Queue"=w1696:refnum<queue>)  [unwired: 7 in]
      }
      event "calculate rotary": Value Change {
        n1103 = event-data() -> ()  [unwired: 1 in, 1 out]
